vi "Sum 4D to 2D.vi"(1 "Array 4D":i32[][][][](array[numeric])) -> (0 "Array 2D":i32[][](array[numeric]))   [LabVIEW 2009]
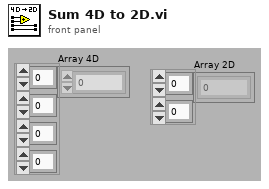
[diagram p1: front panel]
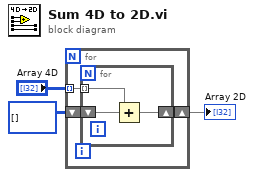
[diagram p0: block diagram]
diagram:
  n1 = for {
    tunnel: "Array 4D" -> [w6] mode=indexing
    shift-right: [w4] -> w1
    shift-left: i32[][] [] -> [w5]
    n2 = for {
      tunnel: w6 -> [w7] mode=indexing
      shift-right: [w8] -> w4
      shift-left: w5 -> [w9]
      n3 = Add(x=w7, y=w9) -> (x+y=w8:i32[][])
    }
  }
  "Array 2D" <- w1
